vi "Legend Pie Prefix.vi"() -> (2 "Prefix Out":string=" ")   [LabVIEW 2017, in "3D Pie.lvclass"]
uses:
  <vilib>/Math Plots/3D Math Plots/3D Pie/3D Pie/3D Pie.lvclass
panel:
  in  "Prefix":string="Slice "
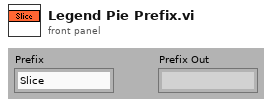
[diagram p1: front panel]
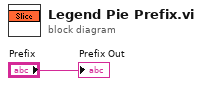
[diagram p0: block diagram]
diagram:
  "Prefix Out" <- "Prefix"
